vi "Call CAL Test.vi"(3 "error in (no error)":errorcluster, 5 "VISA resource name":refnum<visa-resource-name>) -> (0 "error out":errorcluster, 1 "Cal Data":T1={"Time"="20:36:08", "Consecutive good readings"=4, "Total readings"=-1, "A/D counts Sensor 1"=3314.919, "A/D counts Sensor 2"=3314.935, "Diff current/previous Sensor 1"=-0.155, "Diff current/previous Sensor 2"=-0.099}, 2 "VISA resource name out":refnum<visa-resource-name>)   [LabVIEW 2012]
panel:
  in  "Delay Time (s)":dbl=5.0
  out "Readings":i32=40
  in  "stop":bool
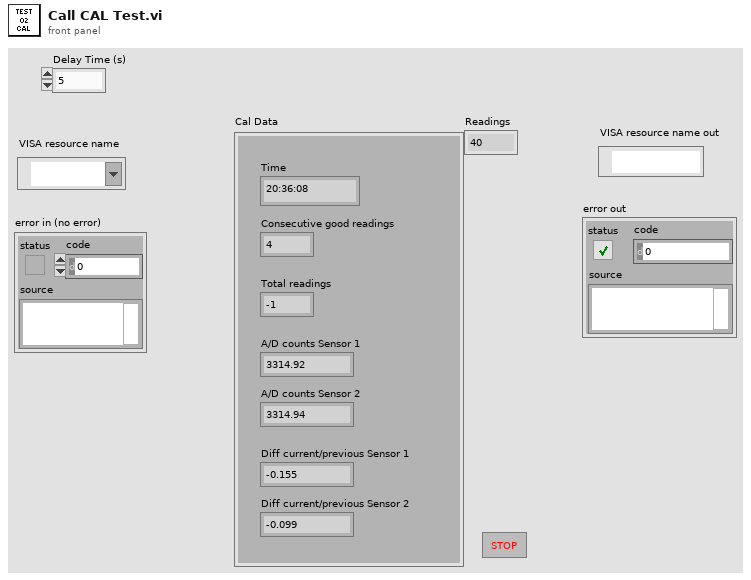
[diagram p1: front panel]
types:
  T1 = cluster{"Time":string, "Consecutive good readings":i32, "Total readings":i32, "A/D counts Sensor 1":sgl, "A/D counts Sensor 2":sgl, "Diff current/previous Sensor 1":sgl, "Diff current/previous Sensor 2":sgl}
  T2 = cluster{"Time":string, "Consecutive good readings":i32, "Total good readings":i32, "A/D counts Sensor 1":sgl, "A/D counts Sensor 2":sgl, "Diff current/previous Sensor 1":sgl, "Diff current/previous Sensor 2":sgl}
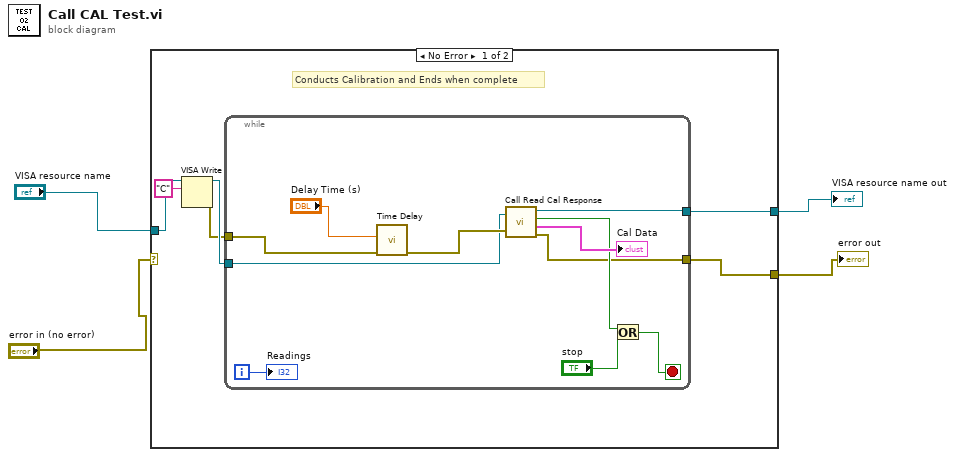
[diagram p0: block diagram]
diagram:
  n1 = case shown="No Error" "error in (no error)" {
    selector: "error in (no error)" -> [_ w22]
    tunnel: "VISA resource name" -> [w8 w23]
    tunnel: [w10 w22] -> w3
    tunnel: [w9 w23] -> w2
    frame No Error {
      # "Conducts Calibration and Ends when complete"
      n2 = VISA Write(VISA resource name=w8, write buffer="C") -> (VISA resource name out=w6:refnum<visa-resource-name>, error out=w5:errorcluster)  [unwired: 1 in, 1 out]
      n3 = while {
        tunnel: w5 -> [w20]
        tunnel: [w16] -> w10
        tunnel: w6 -> [w12]
        tunnel: [w11] -> w9
        i -> [w15]
        stop <- w14 stop-if-true
        n4 = call "Time Delay"("error in (no error)"=w20, "Delay Time (s)"="Delay Time (s)") -> ("error out"=w21:errorcluster)  [unwired: 9 in]
        n5 = call "Call Read Cal Response.vi"("Port"=w12, "error in"=w21) -> ("VISA resource name out"=w11:refnum<visa-resource-name>, "CAL Complete"=w17:bool, "Cal Data"=→"Cal Data":T2, "error out"=w16:errorcluster)
        n6 = Or(x=w17, y="stop") -> (x .or. y?=w14:bool)
        "Readings" <- w15
      }
    }
    frame Error {
    }
  }
  "error out" <- w3
  "VISA resource name out" <- w2
